vi "Read Observation.vi"(8 "error in (no error)":errorcluster, 11 "ObserverRegistryCommand.lvclass in":refnum<class "ObserverRegistryCommand.lvclass">) -> (0 "error out":errorcluster, 2 "Observer":refnum<class "Send.lvclass">, 3 "ObserverRegistryCommand.lvclass out":refnum<class "ObserverRegistryCommand.lvclass">)   [LabVIEW 2011, in "Messenging.lvlib" / "ObserverRegistryCommand.lvclass"]
uses:
  ObserverRegistryCommand.lvclass
  Interprocess Messenger/Send/Send.lvclass
  ObserverRegistryCommand.lvclass/ObserverRegistryCommand.ctl
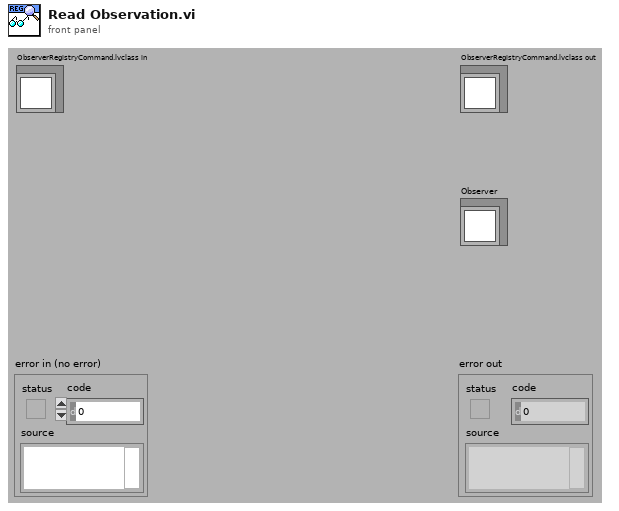
[diagram p1: front panel]
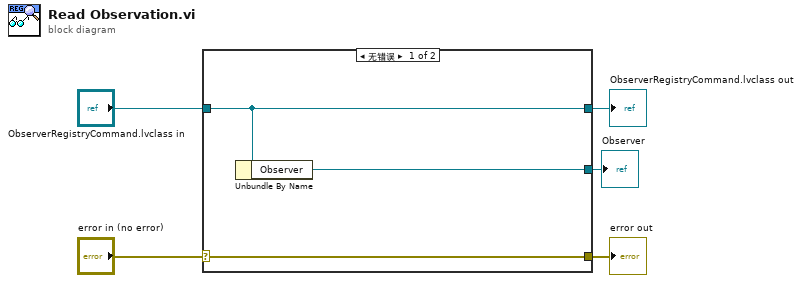
[diagram p0: block diagram]
diagram:
  n1 = case shown="无错误" "error in (no error)" {
    selector: "error in (no error)" -> [w8 w9]
    tunnel: [w8 w9] -> w4
    tunnel: [w7 w10] -> w2
    tunnel: "ObserverRegistryCommand.lvclass in" -> [w7 w10]
    tunnel: [w6 _] -> w1
    frame No Error {
      n2 = Unbundle By Name(w7) -> ("Observer"=w6:refnum<class "Send.lvclass">)
    }
    frame Error {
    }
  }
  "error out" <- w4
  "ObserverRegistryCommand.lvclass out" <- w2
  "Observer" <- w1
